vi "Read.vi"(7 "number of samples":i32=500, 8 "error in (no error)":errorcluster, 10 "settling time (s)":dbl=0.002 format="%#_6p", 11 "voltage level (V)":dbl=0.2 format="%#_6p") -> (0 "error out":errorcluster, 1 "current (A)":dbl, 2 "read voltage (V)":dbl, 3 "resistance (ohm)":dbl format="%#_6p")   [LabVIEW 2019]
uses:
  Globals.vi
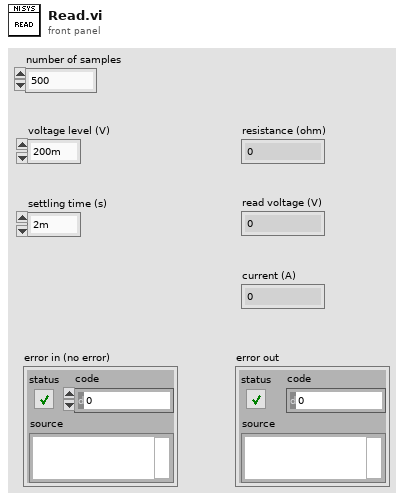
[diagram p1: front panel]
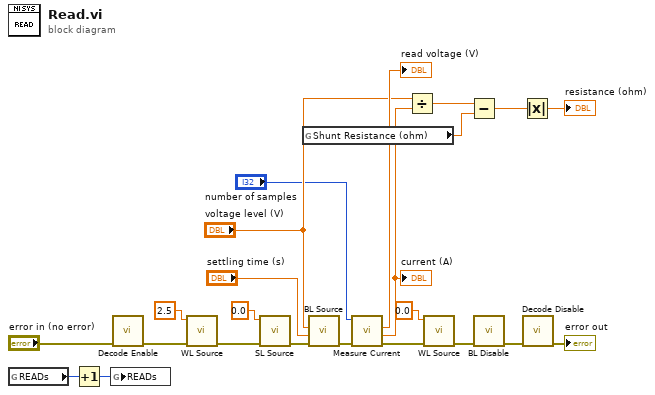
[diagram p0: block diagram]
diagram:
  n1 = global read "Globals.vi" "READs"() -> (w23:u32)
  n2 = Increment(x=w23) -> (x+1=w22:u32)
  n3 = global write "Globals.vi" "READs"(w22) -> ()
  n4 = call "Decode Enable.vi"("error in (no error)"="error in (no error)") -> ("error out"=w12:errorcluster)  [unwired: 10 in]
  n5 = call "WL Source.vi"("error in (no error)"=w12, "VWL (V)"=2.5) -> ("error out"=w3:errorcluster)  [unwired: 9 in]
  n6 = call "SL Source.vi"("error in (no error)"=w3, "voltage level (V)"=0.0 ("SL Voltage (V)")) -> ("error out"=w2:errorcluster)  [unwired: 9 in]
  n7 = global read "Globals.vi" "Shunt Resistance (ohm)"() -> (w7:dbl)
  n8 = call "BL Source.vi"("error in (no error)"=w2, "settling time (s)"="settling time (s)", "voltage level (V)"="voltage level (V)") -> ("error out"=w17:errorcluster)  [unwired: 8 in]
  n9 = call "Measure Current.vi"("error in (no error)"=w17, "number of samples"="number of samples") -> ("error out"=w6:errorcluster, "read current (A)"=w19:dbl, "read voltage (V)"=→"read voltage (V)":dbl)  [unwired: 7 in]
  "current (A)" <- w19
  n10 = Divide(x="voltage level (V)", y=w19) -> (x/y=w9:dbl)
  n11 = call "WL Source.vi"("error in (no error)"=w6, "VWL (V)"=0.0) -> ("error out"=w5:errorcluster)  [unwired: 9 in]
  n12 = Subtract(x=w9, y=w7) -> (x-y=w8:dbl)
  n13 = call "BL Disable.vi"("error in (no error)"=w5) -> ("error out"=w14:errorcluster)  [unwired: 10 in]
  n14 = Absolute Value(x=w8) -> (abs(x)=→"resistance (ohm)":dbl)
  n15 = call "Decode Disable.vi"("error in (no error)"=w14) -> ("error out"=→"error out":errorcluster)  [unwired: 10 in]
